vi "Symphony ProcessDat.vi"(4 "Window Width (ds)":dbl format="%#_13g", 6 "Avg Samples":u32, 7 "Noise Window":bool, 8 "error in (no error)":errorcluster caption="entrée d'erreur (pas d'erreur)", 9 "Noise Substract":T1, 10 "Image Mode":bool, 11 "RawDataIn":i32[][][](array[numeric])) -> (0 "error out":errorcluster caption="sortie d'erreur", 3 "TableauOut":dbl[][](array[numeric]))   [LabVIEW 2019]
uses:
  <userlib>/JY Symphony/NoiseCorr.ctl
panel:
  out "Column":i32
  out "Row":i32
  out "Page":i32
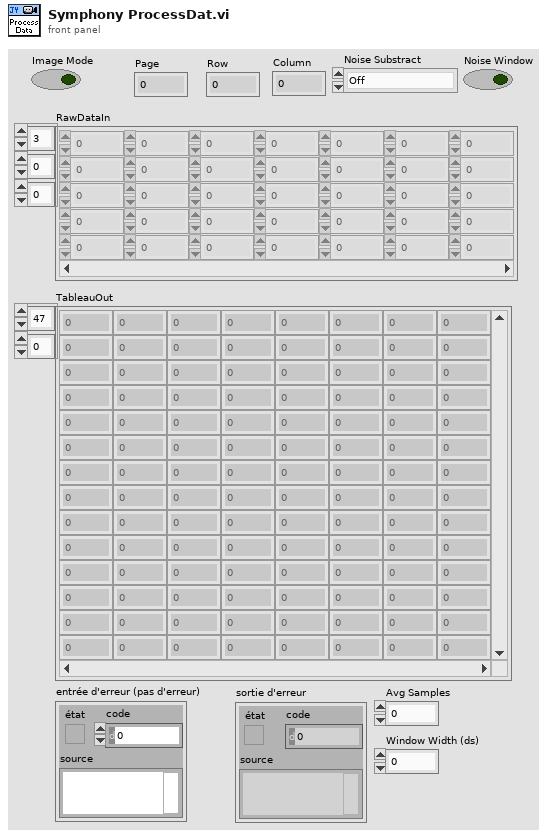
[diagram p1: front panel]
types:
  T1 = typedef "NoiseCorr.ctl" = enum16{"Off", "One For All Acq", "One For Every Acq"}
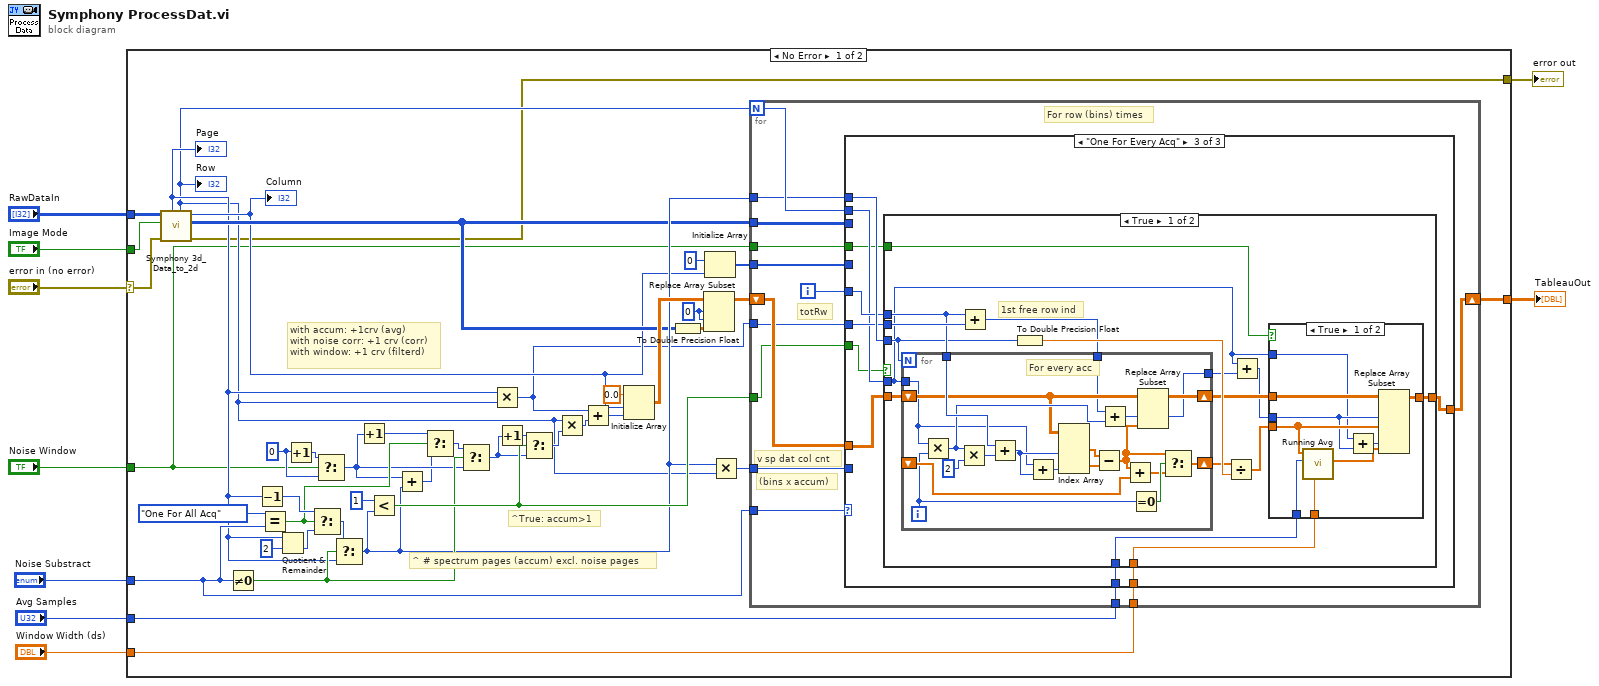
[diagram p0: block diagram]
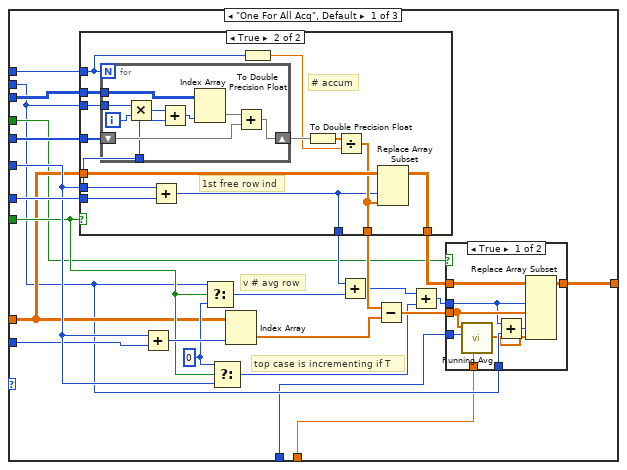
[diagram p2: hidden frame]
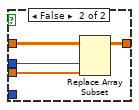
[diagram p3: hidden frame]
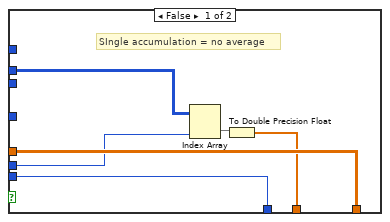
[diagram p4: hidden frame]
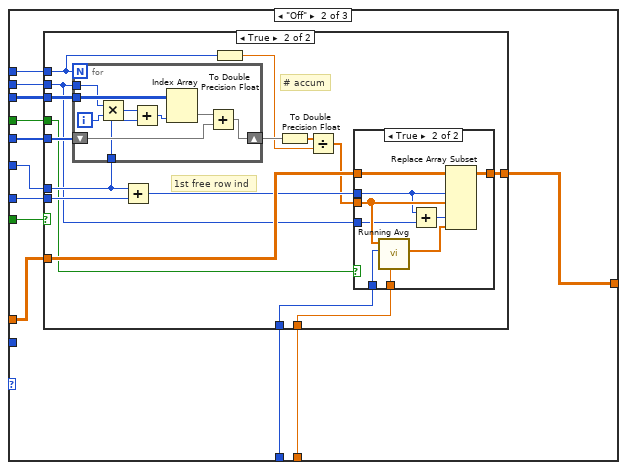
[diagram p5: hidden frame]
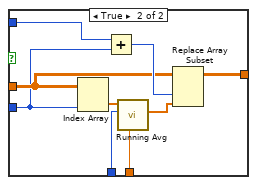
[diagram p7: hidden frame]
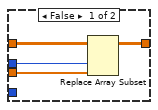
[diagram p8: hidden frame]
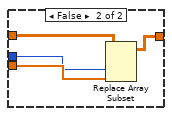
[diagram p9: hidden frame]
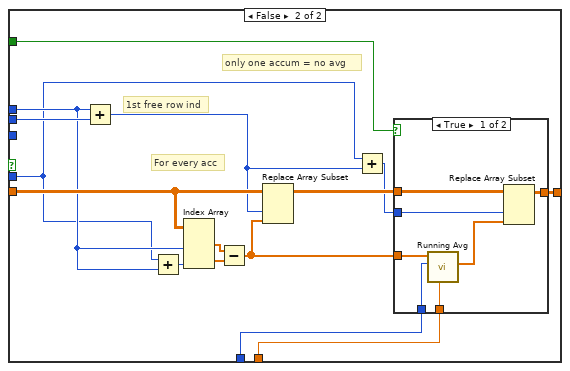
[diagram p10: hidden frame]
diagram:
  n1 = case shown="No Error" "error in (no error)" {
    selector: "error in (no error)" -> [w14 w280]
    tunnel: "Image Mode" -> [w18 _]
    tunnel: "RawDataIn" -> [w21 _]
    tunnel: [w46 _] -> w7
    tunnel: [w13 w280] -> w5
    tunnel: "Noise Substract" -> [w32 _]
    tunnel: "Noise Window" -> [w12 _]
    tunnel: "Avg Samples" -> [w11 _]
    tunnel: "Window Width (ds)" -> [w10 _]
    frame No Error {
      w37 = 0 ("y")
      w47 = 0 ("indice (ligne)")
      # "^True: accum>1"
      # "with accum: +1crv (avg)\nwith noise corr: +1 crv (corr)\nwith window: +1 crv (filterd)"
      # "^ # spectrum pages (accum) excl. noise pages"
      n2 = call <userlib>:"Symphony 3d_Data_to_2d.vi"("error in (no error)"=w14, "Image Mode"=w18, "RawDataIn"=w21) -> ("error out"=w13:errorcluster, "RawDataOut"=w20:i32[][], "Column"=w19:i32, "Row"=w15:i32, "Page"=w17:i32)  [unwired: 4 in]
      "Page" <- w17
      "Row" <- w15
      "Column" <- w19
      n3 = Not Equal To 0?(x=w32) -> (x != 0?=w34:bool)
      n4 = Decrement(x=w17) -> (x-1=w31:i32)
      n5 = Equal?(x=NoiseCorr."One For All Acq" ("Noise Substract"), y=w32) -> (x = y?=w27:bool)
      n6 = Quotient & Remainder(x=w17, y=2) -> (floor(x/y)=w28:i32)  [unwired: 1 out]
      n7 = Increment(x=w37) -> (x+1=w38:i32)
      n8 = Select(t=w31, s=w27, f=w28) -> (s? t:f=w29:i32)
      n9 = Select(t=w38, s=w12, f=w37) -> (s? t:f=w24:i32)
      n10 = Select(t=w29, s=w34, f=w17) -> (s? t:f=w25:i32)
      n11 = Increment(x=w24) -> (x+1=w26:i32)
      n12 = Less?(x=1 ("y"), y=w25) -> (x < y?=w39:bool)
      n13 = Add(x=w24, y=w25) -> (x+y=w23:i32)
      n14 = Select(t=w26, s=w27, f=w23) -> (s? t:f=w22:i32)
      n15 = Select(t=w22, s=w34, f=w24) -> (s? t:f=w36:i32)
      n16 = Multiply(x=w17, y=w15) -> (x*y=w16:i32)
      n17 = Increment(x=w36) -> (x+1=w35:i32)
      n18 = Select(t=w35, s=w39, f=w36) -> (s? t:f=w43:i32)
      n19 = Multiply(x=w15, y=w43) -> (x*y=w44:i32)
      n20 = Add(x=w16, y=w44) -> (x+y=w49:i32)
      n21 = Initialize Array(0.0 ("élément"), w19, w49) -> (w48:dbl[][])
      n22 = To Double Precision Float(number=w20) -> (double precision float=w45:dbl[][])
      n23 = Replace Array Subset(array=w48, new element=w45, index (row)=w47, index (col)=w47) -> (w42:dbl[][])
      n24 = Initialize Array(0 ("élément"), w19) -> (w51:i32[])
      n25 = Multiply(x=w25, y=w15) -> (x*y=w41:i32)
      n26 = for {
        N: w15 -> [w61]
        tunnel: w25 -> [w60]
        tunnel: w16 -> [w63]
        tunnel: w51 -> [w65]
        shift-right: [w62] -> w46
        shift-left: w42 -> [w64]
        tunnel: w20 -> [w66]
        tunnel: w41 -> [w56]
        tunnel: w32 -> [w57]
        tunnel: w39 -> [w58]
        tunnel: w12 -> [w55]
        tunnel: w11 -> [w54]
        tunnel: w10 -> [w53]
        i -> [w59]
        # "(bins x accum)"
        # "For row (bins) times"
        # "v sp dat col cnt"
        # "totRw"
        n27 = case shown="\"One For Every Acq\"" w57 {
          tunnel: w66 -> [w90 w143 _]
          tunnel: w65 -> [w89 w142 _]
          tunnel: w64 -> [w71 w137 w206]
          tunnel: w63 -> [w88 w141 w207]
          tunnel: [w85 w136 w204] -> w62
          tunnel: w61 -> [w69 w135 w203]
          tunnel: w60 -> [w83 w140 w208]
          tunnel: w59 -> [w82 w139 w205]
          tunnel: w56 -> [w81 _ _]
          tunnel: w58 -> [w72 w138 w199]
          tunnel: w55 -> [w70 w134 w202]
          tunnel: w54 -> [w67 w133 w201]
          tunnel: w53 -> [w68 w132 w200]
          frame "One For All Acq", Default {
            w74 = 0 ("f")
            # "top case is incrementing if T"
            # "v # avg row"
            n28 = case shown="True" w72 {
              tunnel: w90 -> [w107 w122]
              tunnel: w89 -> [_ w120]
              tunnel: w83 -> [_ w110]
              tunnel: w71 -> [w109 w117]
              tunnel: w88 -> [w108 w116]
              tunnel: w82 -> [w104 w115]
              tunnel: [w105 w114] -> w87
              tunnel: [w109 w113] -> w86
              tunnel: [w108 w112] -> w84
              tunnel: w69 -> [_ w111]
              frame False {
                # "SIngle accumulation = no average"
                n29 = Index Array(array=w107, index (col)=w104) -> (element=w106:i32[])  [unwired: 1 in]
                n30 = To Double Precision Float(number=w106) -> (double precision float=w105:dbl[])
              }
              frame True {
                # "1st free row ind"
                # "# accum"
                n31 = for {
                  N: w110 -> [_]
                  tunnel: w111 -> [w129]
                  tunnel: w115 -> [w123]
                  shift-right: [w125] -> w121
                  shift-left: w120 -> [w124]
                  tunnel: w122 -> [w130]
                  i -> [w131]
                  n32 = Multiply(x=w129, y=w131) -> (x*y=w128:i32)
                  n33 = Add(x=w128, y=w123) -> (x+y=w127:i32)
                  n34 = Index Array(array=w130, index (col)=w127) -> (element=w126:i32[])  [unwired: 1 in]
                  n35 = Add(x=w126, y=w124) -> (x+y=w125:i32[])
                }
                n36 = Add(x=w115, y=w116) -> (x+y=w112:i32)
                n37 = To Double Precision Float(number=w110) -> (double precision float=w118:dbl)
                n38 = To Double Precision Float(number=w121) -> (double precision float=w119:dbl[])
                n39 = Divide(x=w119, y=w118) -> (x/y=w114:dbl[])
                n40 = Replace Array Subset(array=w117, new element=w114, index (col)=w112) -> (w113:dbl[][])  [unwired: 1 in]
              }
            }
            n41 = Add(x=w82, y=w81) -> (x+y=w80:i32)
            n42 = Select(t=w69, s=w72, f=w74) -> (s? t:f=w77:i32)
            n43 = Select(t=w74, s=w72, f=w82) -> (s? t:f=w73:i32)
            n44 = Index Array(array=w71, index (col)=w80) -> (element=w79:dbl[])  [unwired: 1 in]
            n45 = Add(x=w84, y=w77) -> (x+y=w76:i32)
            n46 = Subtract(x=w87, y=w79) -> (x-y=w78:dbl[])
            n47 = Add(x=w76, y=w73) -> (x+y=w75:i32)
            n48 = case shown="True" w70 {
              tunnel: w86 -> [w99 w103]
              tunnel: [w98 w102] -> w85
              tunnel: w78 -> [w97 w101]
              tunnel: w75 -> [w96 w100]
              tunnel: w69 -> [w94 _]
              tunnel: w67 -> [w92 _]
              tunnel: w68 -> [w91 _]
              frame True {
                n49 = call <userlib>:"Running Avg.vi"("Window Width (ds)"=w91, "Samples cnt"=w92, "Data In"=w97) -> ("Corrected"=w93:dbl[])  [unwired: 6 in, 2 out]
                n50 = Add(x=w96, y=w94) -> (x+y=w95:i32)
                n51 = Replace Array Subset(array=w99, new element #1=w97, index (col) #1=w96, new element #2=w93, index (col) #2=w95) -> (w98:dbl[][])  [unwired: 2 in]
              }
              frame False {
                n52 = Replace Array Subset(array=w103, new element=w101, index (col)=w100) -> (w102:dbl[][])  [unwired: 1 in]
              }
            }
          }
          frame "Off" {
            n53 = case shown="True" w138 {
              tunnel: w143 -> [_ w176]
              tunnel: w142 -> [_ w174]
              tunnel: w140 -> [_ w164]
              tunnel: w137 -> [w150 w171]
              tunnel: w141 -> [_ w170]
              tunnel: w139 -> [w148 w167]
              tunnel: [w147 w169] -> w136
              tunnel: w135 -> [w149 w161]
              tunnel: w134 -> [w146 w165]
              tunnel: w133 -> [w144 w163]
              tunnel: w132 -> [w145 w162]
              frame False {
                # "SIngle accumulation = no average"
                n54 = case shown="False" w146 {
                  tunnel: w150 -> [w151 w156]
                  tunnel: w149 -> [_ w159]
                  tunnel: w148 -> [_ w155]
                  tunnel: [w151 w157] -> w147
                  tunnel: w145 -> [_ w152]
                  tunnel: w144 -> [_ w153]
                  frame False {
                  }
                  frame True {
                    n55 = Index Array(array=w156, index (col)=w155) -> (element=w160:dbl[])  [unwired: 1 in]
                    n56 = Add(x=w159, y=w155) -> (x+y=w158:i32)
                    n57 = call <userlib>:"Running Avg.vi"("Window Width (ds)"=w152, "Samples cnt"=w153, "Data In"=w160) -> ("Corrected"=w154:dbl[])  [unwired: 6 in, 2 out]
                    n58 = Replace Array Subset(array=w156, new element=w154, index (col)=w158) -> (w157:dbl[][])  [unwired: 1 in]
                  }
                }
              }
              frame True {
                # "1st free row ind"
                # "# accum"
                n59 = for {
                  N: w164 -> [_]
                  tunnel: w161 -> [w196]
                  tunnel: w167 -> [w190]
                  shift-right: [w192] -> w175
                  shift-left: w174 -> [w191]
                  tunnel: w176 -> [w197]
                  i -> [w198]
                  n60 = Multiply(x=w196, y=w198) -> (x*y=w195:i32)
                  n61 = Add(x=w195, y=w190) -> (x+y=w194:i32)
                  n62 = Index Array(array=w197, index (col)=w194) -> (element=w193:i32[])  [unwired: 1 in]
                  n63 = Add(x=w193, y=w191) -> (x+y=w192:i32[])
                }
                n64 = Add(x=w167, y=w170) -> (x+y=w168:i32)
                n65 = To Double Precision Float(number=w164) -> (double precision float=w172:dbl)
                n66 = To Double Precision Float(number=w175) -> (double precision float=w173:dbl[])
                n67 = Divide(x=w173, y=w172) -> (x/y=w166:dbl[])
                n68 = case shown="True" w165 {
                  tunnel: w171 -> [w180 w189]
                  tunnel: [w179 w188] -> w169
                  tunnel: w168 -> [w178 w186]
                  tunnel: w166 -> [w177 w187]
                  tunnel: w161 -> [_ w185]
                  tunnel: w163 -> [_ w182]
                  tunnel: w162 -> [_ w181]
                  frame False {
                    n69 = Replace Array Subset(array=w180, new element=w177, index (col)=w178) -> (w179:dbl[][])  [unwired: 1 in]
                  }
                  frame True {
                    n70 = call <userlib>:"Running Avg.vi"("Window Width (ds)"=w181, "Samples cnt"=w182, "Data In"=w187) -> ("Corrected"=w183:dbl[])  [unwired: 6 in, 2 out]
                    n71 = Add(x=w186, y=w185) -> (x+y=w184:i32)
                    n72 = Replace Array Subset(array=w189, new element #1=w187, index (col) #1=w186, new element #2=w183, index (col) #2=w184) -> (w188:dbl[][])  [unwired: 2 in]
                  }
                }
              }
            }
          }
          frame "One For Every Acq" {
            n73 = case shown="True" w199 {
              tunnel: w208 -> [w210 _]
              tunnel: w207 -> [w223 w271]
              tunnel: w206 -> [w222 w270]
              tunnel: w205 -> [w220 w259]
              tunnel: [w218 w268] -> w204
              tunnel: w203 -> [w209 w258]
              tunnel: w202 -> [w213 w266]
              tunnel: w201 -> [w212 w265]
              tunnel: w200 -> [w211 w264]
              frame True {
                # "1st free row ind"
                n74 = Add(x=w220, y=w223) -> (x+y=w221:i32)
                n75 = for {
                  N: w210 -> [_]
                  tunnel: w220 -> [w255]
                  tunnel: w221 -> [w245]
                  tunnel: w209 -> [w244]
                  shift-right: [w256] -> w219
                  shift-left: w222 -> [w247]
                  shift-right: [w242] -> w216
                  shift-left: _ -> [w246]
                  tunnel: [w243] -> w214
                  i -> [w241]
                  # "For every acc"
                  n76 = Multiply(x=w244, y=w241) -> (x*y=w248:i32)
                  n77 = Multiply(x=w248, y=2) -> (x*y=w250:i32)
                  n78 = Add(x=w255, y=w250) -> (x+y=w253:i32)
                  n79 = Add(x=w244, y=w253) -> (x+y=w254:i32)
                  n80 = Index Array(array=w247, index (col) #1=w253, index (col) #2=w254) -> (element #1=w252:dbl[], element #2=w251:dbl[])  [unwired: 2 in]
                  n81 = Subtract(x=w252, y=w251) -> (x-y=w239:dbl[])
                  n82 = Add(x=w245, y=w248) -> (x+y=w243:i32)
                  n83 = Add(x=w239, y=w246) -> (x+y=w238:dbl[])
                  n84 = Equal To 0?(x=w241) -> (x = 0?=w240:bool)
                  n85 = Replace Array Subset(array=w247, new element=w239, index (col)=w243) -> (w256:dbl[][])  [unwired: 1 in]
                  n86 = Select(t=w239, s=w240, f=w238) -> (s? t:f=w242:dbl[])
                }
                n87 = To Double Precision Float(number=w210) -> (double precision float=w224:dbl)
                n88 = Divide(x=w216, y=w224) -> (x/y=w217:dbl[])
                n89 = Add(x=w209, y=w214) -> (x+y=w215:i32)
                n90 = case shown="True" w213 {
                  tunnel: w219 -> [w233 w237]
                  tunnel: [w232 w236] -> w218
                  tunnel: w217 -> [w231 w235]
                  tunnel: w215 -> [w230 w234]
                  tunnel: w209 -> [w227 _]
                  tunnel: w212 -> [w226 _]
                  tunnel: w211 -> [w225 _]
                  frame True {
                    n91 = call <userlib>:"Running Avg.vi"("Window Width (ds)"=w225, "Samples cnt"=w226, "Data In"=w231) -> ("Corrected"=w228:dbl[])  [unwired: 6 in, 2 out]
                    n92 = Add(x=w227, y=w230) -> (x+y=w229:i32)
                    n93 = Replace Array Subset(array=w233, new element #1=w231, index (col) #1=w230, new element #2=w228, index (col) #2=w229) -> (w232:dbl[][])  [unwired: 2 in]
                  }
                  frame False {
                    n94 = Replace Array Subset(array=w237, new element=w235, index (col)=w234) -> (w236:dbl[][])  [unwired: 1 in]
                  }
                }
              }
              frame False {
                # "For every acc"
                # "only one accum = no avg"
                # "1st free row ind"
                n95 = Add(x=w259, y=w271) -> (x+y=w257:i32)
                n96 = Add(x=w258, y=w259) -> (x+y=w262:i32)
                n97 = Index Array(array=w270, index (col) #1=w259, index (col) #2=w262) -> (element #1=w261:dbl[], element #2=w260:dbl[])  [unwired: 2 in]
                n98 = Subtract(x=w261, y=w260) -> (x-y=w263:dbl[])
                n99 = Replace Array Subset(array=w270, new element=w263, index (col)=w257) -> (w269:dbl[][])  [unwired: 1 in]
                n100 = Add(x=w258, y=w257) -> (x+y=w267:i32)
                n101 = case shown="True" w266 {
                  tunnel: w269 -> [w278 w279]
                  tunnel: [w277 w279] -> w268
                  tunnel: w263 -> [w276 _]
                  tunnel: w267 -> [w275 _]
                  tunnel: w265 -> [w274 _]
                  tunnel: w264 -> [w273 _]
                  frame True {
                    n102 = call <userlib>:"Running Avg.vi"("Window Width (ds)"=w273, "Samples cnt"=w274, "Data In"=w276) -> ("Corrected"=w272:dbl[])  [unwired: 6 in, 2 out]
                    n103 = Replace Array Subset(array=w278, new element=w272, index (col)=w275) -> (w277:dbl[][])  [unwired: 1 in]
                  }
                  frame False {
                  }
                }
              }
            }
          }
        }
      }
    }
    frame Error {
    }
  }
  "TableauOut" <- w7
  "error out" <- w5
